vi "read n bytes from internal stream.vi"(8 "error in":errorcluster, 9 "length":u64, 11 "connection in":refnum<class "connection.lvclass">) -> (0 "error out":errorcluster, 3 "buffer":string)   [LabVIEW 2016, in "connection.lvclass"]
uses:
  connection.lvclass
  connection.lvclass/connection.ctl
  dllwrapper/library path.vi
  <vilib>/Utility/error.llb/Error Cluster From Error Code.vi
  dllwrapper/async tls dl.lvlib
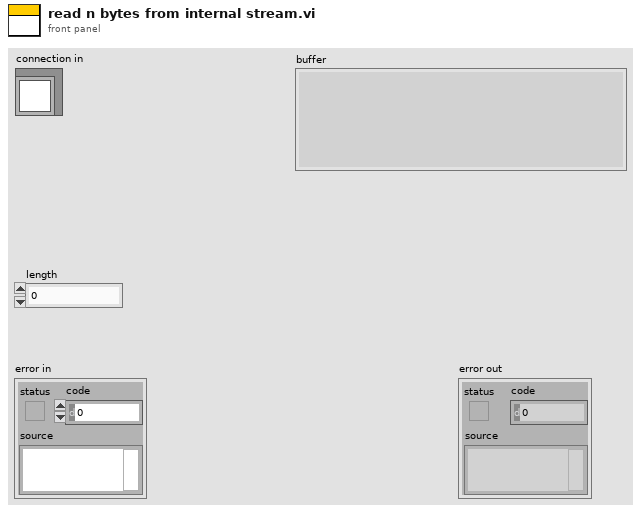
[diagram p1: front panel]
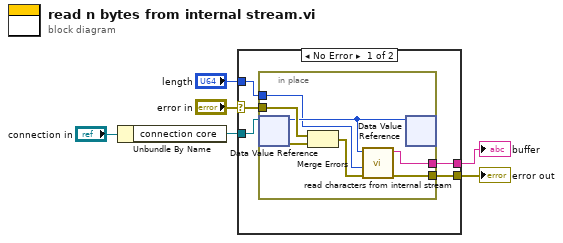
[diagram p0: block diagram]
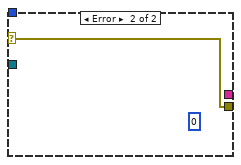
[diagram p2: hidden frame]
diagram:
  n1 = Unbundle By Name("connection in") -> ("connection core"=w5:refnum<data-value>)
  n2 = case shown="No Error" "error in" {
    selector: "error in" -> [w10 w19]
    tunnel: w5 -> [w11 _]
    tunnel: [w9 w19] -> w3
    tunnel: [w8 _] -> w2
    tunnel: "length" -> [w7 _]
    frame No Error {
      n3 = in-place {
        in-place-border: w10 -> [w18]
        in-place-border: [w15] -> w9
        in-place-border: [w13] -> w8
        in-place-border: w7 -> [w12]
        n4 = in-place-dvr #1(w11) -> (w14:u64, w17:errorcluster)
        n5 = Merge Errors(w18, w17) -> (w16:errorcluster)
        n6 = call "read characters from internal stream.vi"("error in"=w16, "length"=w12, "socket"=w14) -> ("error out"=w15:errorcluster, "buffer"=w13:string)  [unwired: 7 in]
        n7 = in-place-dvr #1(w14) -> ()  [unwired: 2 out]
      }
    }
    frame Error {
      (unwired) u64 0 ("size")
    }
  }
  "error out" <- w3
  "buffer" <- w2
